vi "WFS Take Spotfield Image.vi"(8 "error in (no error)":errorcluster {"code" format="%.0x"}, 11 "instrument handle":refnum<visa-resource-name>) -> (0 "error out":errorcluster {"code" format="%.0x"}, 3 "instrument handle out":refnum<visa-resource-name>)   [LabVIEW 2020]
doc: "This VI receives a spotfield image from the WFS camera into a driver buffer. The reference to this buffer is provided by VI GetSpotfieldImage() and an image copy is returned by VI GetSpotfieldImageCopy().\n\nIn case of unsuited image exposure the VI sets the appropriate status bits. Use VI GetStatus() to check the reason.\n\nBit Name Meaning if bit is set\n\n0x00000002 WFS_STATBIT_PTH (2) Power Too High (cam saturated)\n0x00000004 WFS_STATBIT_PTL (4) Power Too Low (low cam digits)\n0x00000008 WFS_STATBIT_HAL (8) High Ambient Light\n\nYou need to set optimized exposure and gain settings by VIs SetExposureTime() and SetMasterGain() and repeate calling the VI until these status bits are cleared.\n\nAlternatively, you may use VI GetImageAutoExpos().\n\n\nWhen the trigger capability is activated by VI SetTriggerMode() this VI will wait for a trigger event for a short period of time (WFS_TIMEOUT_CAPTURE_TRIGGER (0.1) = 0.1 sec.) prior to start exposure and will return with error WFS_ERROR_AWAITING_TRIGGER (-1074001642) if no trigger event occured.\nYou need to repeate calling this VI until this error and status bit WFS_STATBIT_ATR (128) disappear."
uses:
  WFS_32.dll
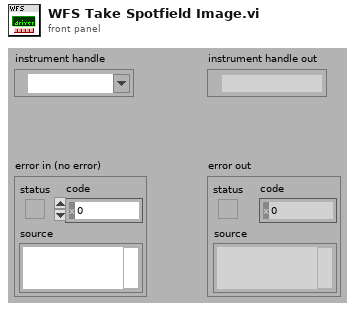
[diagram p1: front panel]
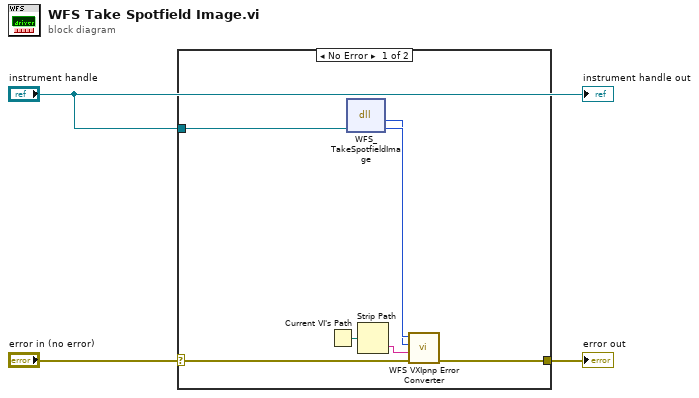
[diagram p0: block diagram]
diagram:
  n1 = case shown="No Error" "error in (no error)" {
    selector: "error in (no error)" -> [w5 w11]
    tunnel: [w4 w11] -> w3
    tunnel: "instrument handle" -> [w9 _]
    frame No Error {
      n2 = Current VI's Path() -> (path=w10:path)
      n3 = dll-call lib="WFS_*.*" fn="WFS_TakeSpotfieldImage"("Instrument Handle"=w9) -> (w7:i32, "Instrument Handle"=w8:u32)  [unwired: 3 in, 2 out]
      n4 = Strip Path(path=w10) -> (name=w6:string)  [unwired: 1 out]
      n5 = call "WFS VXIpnp Error Converter.vi"("error in (no error)"=w5, "Name Of VI (\"\")"=w6, "CVI Error Code (0)"=w7, "instrument handle"=w8) -> ("error out"=w4:errorcluster)  [unwired: 6 in, 1 out]
    }
    frame Error {
    }
  }
  "error out" <- w3
  "instrument handle out" <- "instrument handle"
